vi "Write focus #stepsdone.vi"(8 "error in (no error)":errorcluster, 10 "focus #stepsdone":u32, 11 "TelFocus in":refnum<class "TelFocus.lvclass">) -> (0 "error out":errorcluster, 3 "TelFocus out":refnum<class "TelFocus.lvclass">)   [LabVIEW 2018, in "TelFocus.lvclass"]
uses:
  TelFocus.lvclass
  TelFocus.lvclass/TelFocus.ctl
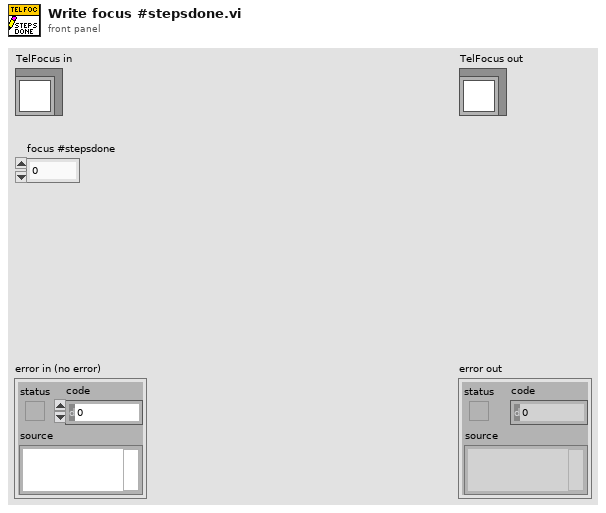
[diagram p1: front panel]
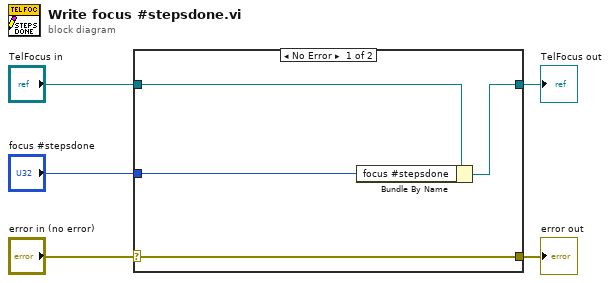
[diagram p0: block diagram]
diagram:
  n1 = case shown="No Error" "error in (no error)" {
    selector: "error in (no error)" -> [w9 w10]
    tunnel: [w9 w10] -> w4
    tunnel: [w7 w11] -> w2
    tunnel: "TelFocus in" -> [w8 w11]
    tunnel: "focus #stepsdone" -> [w6 _]
    frame No Error {
      n2 = Bundle By Name(cluster=w8, "focus #stepsdone"=w6) -> (w7:refnum<class "TelFocus.lvclass">)
    }
    frame Error {
    }
  }
  "error out" <- w4
  "TelFocus out" <- w2
